vi "Fpga-ItchParser.vi"() -> ()   [LabVIEW 2016]
uses:
  <vilib>/Platform/TimedLoop/XDataNode/timing_clust.ctl
  <vilib>/Platform/TimedLoop/XDataNode/nitl_modes.ctl
  <vilib>/Platform/TimedLoop/XDataNode/wakeup.ctl
  <vilib>/rvi/Emulation/niFpgaSctlEmulationGetInTimedLoop.vi
  <vilib>/rvi/Emulation/niFpgaEmulationReportErrorSimple.vi
  <vilib>/rvi/Emulation/niFpgaGetClockAttributes.vi
  <vilib>/rvi/Emulation/niFpgaCriticalErrorInLSC.vi
  <vilib>/rvi/Emulation/niFpgaEmulationIsFPGAContextNoSignature.vi
  <vilib>/rvi/errors/niFpgaSetErrorForExecOnDevCompSimple.vi
  <vilib>/rvi/eio/common/nirviEmuReportErrorAndStop.vi
  <vilib>/rvi/DataTransferAndStorage/Container/Common/niFpgaContainerGetUniqueNameForEmu.vi
  <vilib>/rvi/FIFO/Fifo_Resource/nirvififoEmulationSetSize.vi
  <vilib>/rvi/FIFO/Fifo_Resource/nirviFifoEmulationQueueMgr.vi
  <instcachedir>/0/nirviFifoEmulationQueueMgr_E5CAEC123FF24DC58D834DCA3CDAA9B5.lvgen/nirviFifoEmulationQueueMgr_E5CAEC123FF24DC58D834DCA3CDAA9B5_008.vi
  <vilib>/Utility/error.llb/Clear Errors.vi
  <vilib>/rvi/FIFO/Fifo_Resource/nirvififoEmulationCreateLock.vi
  <vilib>/rvi/Emulation/niFpgaProcessEmulError.vi
  <vilib>/rvi/FIFO/Fifo_Resource/nirvififoEmulationObtainLock.vi
  <vilib>/rvi/FIFO/Fifo_Resource/nirvififoEmulationReleaseLock.vi
  <vilib>/rvi/occurrence/nirviWaitOnOccurrenceBase.vi
  <vilib>/rvi/errors/nirviReportUnexpectedCaseInternalError.vi
  <vilib>/rvi/errors/nirviReportUnexpectedCaseInternalError (U32).vi
  <instcachedir>/0/nirviFifoEmulationQueueMgr_E5CAEC123FF24DC58D834DCA3CDAA9B5.lvgen/nirviFifoEmulationQueueMgr_E5CAEC123FF24DC58D834DCA3CDAA9B5_009.vi
  <vilib>/rvi/FIFO/Fifo_Resource/nirvififoEmulationDetermineInputValidOut.vi
  <vilib>/Platform/TimedLoop/XDataNode/XDataNode.xnode
  <vilib>/rvi/DataTransferAndStorage/Container/XNode/niFpgaContainer.xnode
  <vilib>/rvi/FIFO/Fifo_Resource/nirvififoEmulationRead.vi
  <vilib>/rvi/FIFO/Fifo_Resource/nirvififoEmulationWrite.vi
  <vilib>/Platform/TimedLoop/XDataNode/XDNodeRunTimeDep.lvlib
panel:
  out "Seconds":u32 format="%.0x"
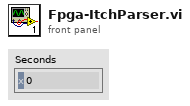
[diagram p1: front panel]
types:
  T1 = cluster{"Operation":enum16{"Noop", "GetAll", "AddOrder", "DeleteOrder"}, "Cluster":cluster{"Side":u16, "OrderRefNum":u64, "Price":u32, "Shares":u32}}
  T2 = typedef "XDNodeRunTimeDep.lvlib/timing_clust.ctl" = cluster{"Expected End [f-1]":u64, "Actual End [f-1]":u64, "Finished Late? [f-1]":bool, "Expected End [i-1]":u64, "Actual End [i-1]":u64, "Finished Late? [i-1]":bool, "Expected Start [i]":u64, "Actual Start [i]":u64, "Expected Start [f]":u64, "Actual Start [f]":u64, "Source Name":string, "Structure Name":string, "Period":i64, "Deadline":i64, "Offset":i64, "Start":i64, "Priority":i32, "Timeout":i32, "Mode":T3, "Wakeup Reason":T4, "Error":errorcluster, "Source Type":string, "Secondary Source Type":string, "Global End Time":u64, "Global Start Time":u64, "Frame Duration":u64, "Iteration Duration":u64, "Assigned CPU":i32, "I/O Scan Engine Mode":u32}
  T3 = typedef "XDNodeRunTimeDep.lvlib/nitl_modes.ctl" = enum32{"No Change", "Process missed periods, maintain original phase", "Discard missed periods, maintain original phase", "Process missed periods, ignore original phase", "Discard missed periods, ignore original phase"}
  T4 = typedef "XDNodeRunTimeDep.lvlib/wakeup.ctl" = enum32{"Normal", "Aborted", "Asynchronous wakeup", "Timing source error", "Timed loop error", "Timeout"}
  T5 = enum16{"Noop", "GetAll", "AddOrder", "DeleteOrder"}
  T6 = cluster{"Side":u16, "OrderRefNum":u64, "Price":u32, "Shares":u32}
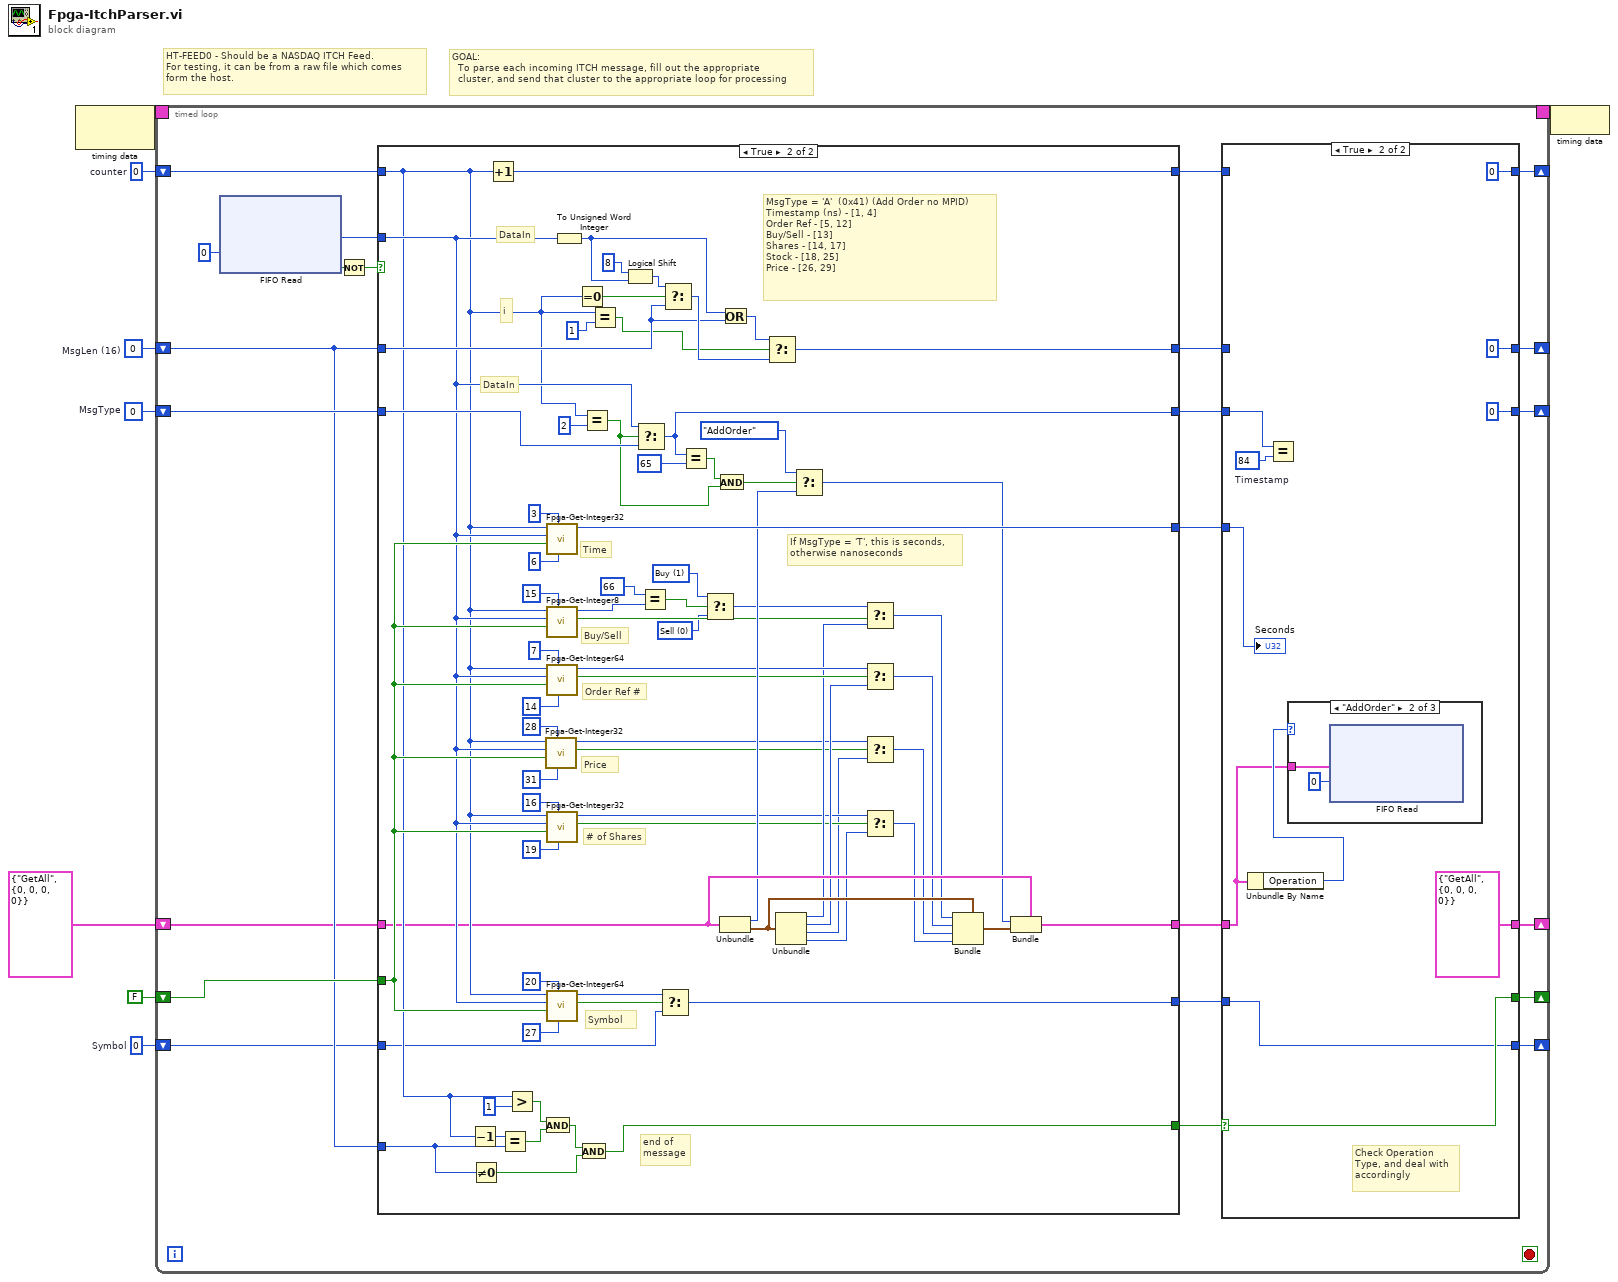
[diagram p0: block diagram]
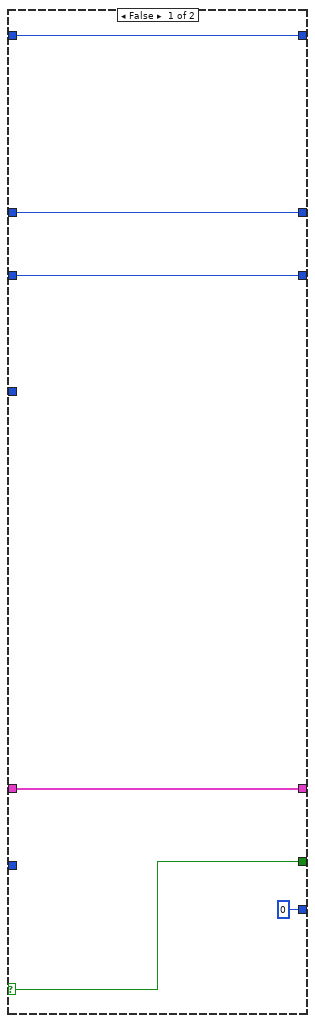
[diagram p2: hidden frame]
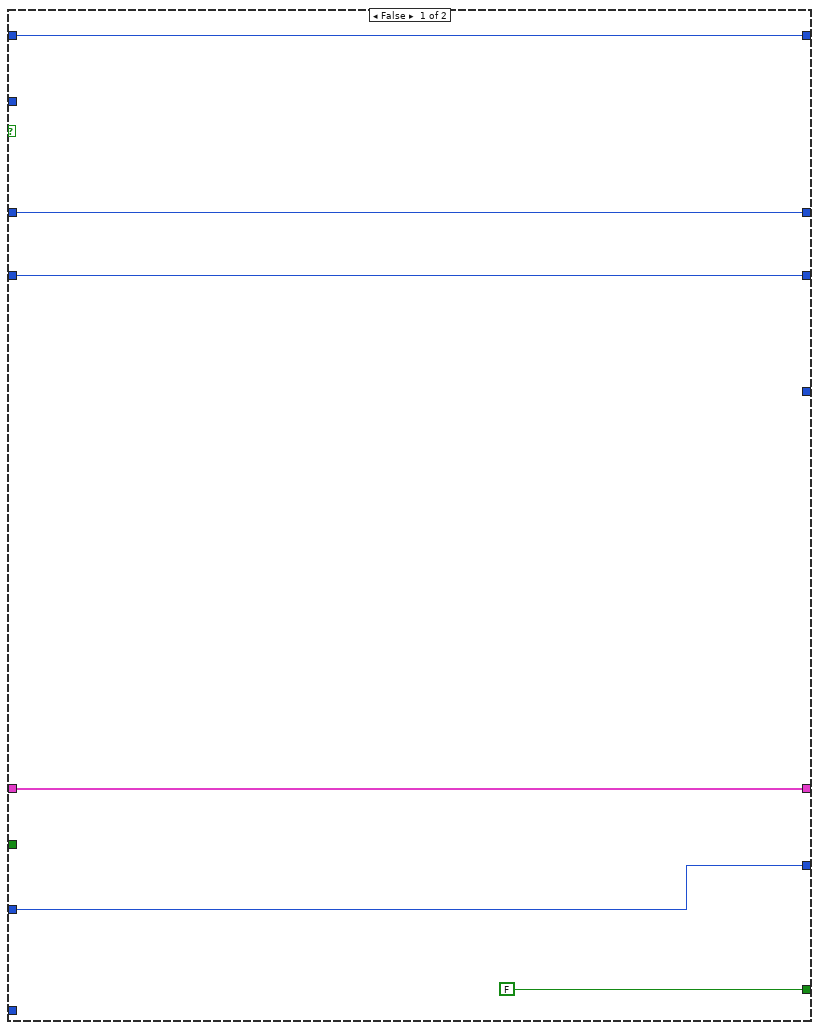
[diagram p5: hidden frame]
diagram:
  w2 = u64 0  # Symbol
  w4 = u8 0  # MsgType
  w5 = u16 0  # counter
  w6 = u16 0  # MsgLen (16)
  # "GOAL:\n  To parse each incoming ITCH message, fill out the appropriate\n  cluster, and send that cluster to the appropriate loop for processing"
  # "HT-FEED0 - Should be a NASDAQ ITCH Feed.\nFor testing, it can be from a raw file which comes\nform the host."
  n1 = node-c288() -> (w8:T2)  [unwired: 1 in]
  n2 = timed-loop {
    timing: w8 -> [_]
    timing-out: [_] -> w7
    shift-right: [w22] -> _
    shift-left: w6 -> [w15]
    shift-right: [w23] -> _
    shift-left: w5 -> [w27]
    shift-right: [w20] -> _
    shift-left: w4 -> [w26]
    shift-right: [w17] -> _
    shift-left: FALSE -> [w16]
    shift-right: [w12] -> _
    shift-left: T1 {"Operation"=enum."GetAll", "Cluster"={"Side"=0, "OrderRefNum"=0, "Price"=0, "Shares"=0}} ("OrderBookCommand") -> [w14]
    shift-right: [w10] -> _
    shift-left: w2 -> [w11]
    stop <- _ stop-if-true
    n3 = xnode ("FIFO Read")("Timeout"=0) -> ("Element"=w28:u8, "Timed Out?"=w30:bool)  [unwired: 1 in, 1 out]
    n4 = Not(x=w30) -> (.not. x?=w29:bool)
    n5 = case shown="True" w29 {
      tunnel: w28 -> [_ w105]
      tunnel: [w56 w125] -> w21
      tunnel: w15 -> [w56 w108]
      tunnel: w27 -> [w55 w104]
      tunnel: [w55 w128] -> w24
      tunnel: w26 -> [w54 w115]
      tunnel: [w54 w86] -> w19
      tunnel: [_ w111] -> w18
      tunnel: [FALSE w112] -> w25
      tunnel: w16 -> [_ w106]
      tunnel: w15 -> [_ w107]
      tunnel: w14 -> [w52 w92]
      tunnel: [w52 w91] -> w13
      tunnel: w11 -> [w51 w61]
      tunnel: [w51 w58] -> w9
      frame False {
      }
      frame True {
        w73 = u16 0 items=["Sell", "Buy"] ("Side")
        w72 = u16 1 items=["Sell", "Buy"] ("Side")
        # "Time"
        # "MsgType = 'A'  (0x41) (Add Order no MPID)\nTimestamp (ns) - [1, 4]\nOrder Ref - [5, 12]\nBuy/Sell - [13]\nShares - [14, 17]\nStock - [18, 25]\nPrice - [26, 29]"
        # "Buy/Sell"
        # "Order Ref #"
        # "# of Shares"
        # "Symbol"
        # "Price"
        # "If MsgType = 'T', this is seconds,\notherwise nanoseconds"
        # "DataIn"
        # "i"
        # "DataIn"
        # "end of\nmessage"
        n6 = Decrement(x=w104) -> (x-1=w117:u16)
        n7 = Not Equal To 0?(x=w107) -> (x != 0?=w114:bool)
        n8 = Increment(x=w104) -> (x+1=w128:u16)
        n9 = Equal?(x=w117, y=w107) -> (x = y?=w118:bool)
        n10 = Greater?(x=w104, y=u16 1) -> (0:w119:bool)
        n11 = And(x=w119, y=w118) -> (x .and. y?=w113:bool)
        n12 = call "Fpga-Get-Integer32.vi"("upper"=u16 31 ("lower"), "lower"=u16 28, "Reset"=w106, "DataIn"=w105, "Index"=w104) -> ("Valid"=w65:bool, "UInt32"=w62:u32)  [unwired: 5 in]
        n13 = call "Fpga-Get-Integer32.vi"("upper"=u16 6, "lower"=u16 3, "Reset"=w106, "DataIn"=w105, "Index"=w104) -> ("UInt32"=w111:u32)  [unwired: 5 in, 1 out]
        n14 = call "Fpga-Get-Integer8.vi"("lower"=u16 15, "Reset"=w106, "DataIn"=w105, "Index"=w104) -> ("Valid"=w77:bool, "U8"=w76:u8)  [unwired: 6 in]
        n15 = call "Fpga-Get-Integer64.vi"("upper"=u16 14 ("lower"), "lower"=u16 7, "Reset"=w106, "DataIn"=w105, "Index"=w104) -> ("Valid"=w82:bool, "UInt32"=w81:u64)  [unwired: 5 in]
        n16 = call "Fpga-Get-Integer32.vi"("upper"=u16 19 ("lower"), "lower"=u16 16, "Reset"=w106, "DataIn"=w105, "Index"=w104) -> ("Valid"=w69:bool, "UInt32"=w68:u32)  [unwired: 5 in]
        n17 = call "Fpga-Get-Integer64.vi"("upper"=u16 27 ("lower"), "lower"=u16 20, "Reset"=w106, "DataIn"=w105, "Index"=w104) -> ("Valid"=w60:bool, "UInt32"=w59:u64)  [unwired: 5 in]
        n18 = To Unsigned Word Integer(number=w105) -> (unsigned 16bit integer=w121:u16)
        n19 = Equal To 0?(x=w104) -> (x = 0?=w127:bool)
        n20 = And(x=w113, y=w114) -> (x .and. y?=w112:bool)
        n21 = Equal?(x=w104, y=u16 2) -> (x = y?=w84:bool)
        n22 = Equal?(x=w104, y=u16 1) -> (x = y?=w90:bool)
        n23 = Logical Shift(y=i16 8, x=w121) -> (x << y=w122:u16)
        n24 = Select(t=w105, s=w84, f=w115) -> (s? t:f=w86:u8)
        n25 = Equal?(x=u8 66, y=w76) -> (x = y?=w74:bool)
        n26 = Select(t=w59, s=w60, f=w61) -> (s? t:f=w58:u64)
        n27 = Select(t=w122, s=w127, f=w108) -> (s? t:f=w126:u16)
        n28 = Equal?(x=w86, y=u8 65) -> (x = y?=w85:bool)
        n29 = Select(t=w72, s=w74, f=w73) -> (s? t:f=w71:u16)
        n30 = And(x=w85, y=w84) -> (x .and. y?=w83:bool)
        n31 = Unbundle(w92) -> ("Operation"=w89:T5, "Cluster"=w94:T6)
        n32 = Or(x=w121, y=w108) -> (x .or. y?=w124:u16)
        n33 = Select(t=w124, s=w90, f=w126) -> (s? t:f=w125:u16)
        n34 = Unbundle(w94) -> ("Side"=w78:u16, "OrderRefNum"=w80:u64, "Price"=w64:u32, "Shares"=w67:u32)
        n35 = Select(t=T5."AddOrder" ("Operation"), s=w83, f=w89) -> (s? t:f=w88:T5)
        n36 = Select(t=w71, s=w77, f=w78) -> (s? t:f=w70:u16)
        n37 = Select(t=w81, s=w82, f=w80) -> (s? t:f=w79:u64)
        n38 = Select(t=w62, s=w65, f=w64) -> (s? t:f=w63:u32)
        n39 = Select(t=w68, s=w69, f=w67) -> (s? t:f=w66:u32)
        n40 = Bundle(cluster=w94, "Side"=w70, "OrderRefNum"=w79, "Price"=w63, "Shares"=w66) -> (w93:T6)
        n41 = Bundle(cluster=w92, "Operation"=w88, "Cluster"=w93) -> (w91:T1)
      }
    }
    n42 = case shown="True" w25 {
      selector: w25 -> [w34 w44]
      tunnel: w24 -> [w35 _]
      tunnel: [w35 u16 0 ("counter")] -> w23
      tunnel: [w36 u16 0 ("MsgLen (16)")] -> w22
      tunnel: w21 -> [w36 _]
      tunnel: [w37 u8 0 ("MsgType")] -> w20
      tunnel: w19 -> [w37 w43]
      tunnel: w18 -> [_ w48]
      tunnel: [w34 w44] -> w17
      tunnel: w13 -> [w33 w38]
      tunnel: [w33 T1 {"Operation"=enum."GetAll", "Cluster"={"Side"=0, "OrderRefNum"=0, "Price"=0, "Shares"=0}} ("OrderBookCommand")] -> w12
      tunnel: [u64 0 ("Symbol") w41] -> w10
      tunnel: w9 -> [_ w41]
      frame False {
      }
      frame True {
        w42 = u8 84  # Timestamp
        # "Check Operation\nType, and deal with\naccordingly"
        n43 = Unbundle By Name(w38) -> ("Operation"=w39:T5)
        n44 = Equal?(x=w43, y=w42) -> ()  [unwired: 1 out]
        n45 = case shown="\"AddOrder\"" w39 {
          tunnel: w38 -> [_ w50 _]
          frame "Noop", Default {
          }
          frame "AddOrder" {
            n46 = xnode ("FIFO Read")("Element"=w50, "Timeout"=0) -> ()  [unwired: 1 in, 2 out]
          }
          frame "DeleteOrder" {
          }
        }
        "Seconds" <- w48
      }
    }
  }
  n47 = node-c288(w7) -> ()
